vi "Configure Offset.vi"(8 "error in (no error)":errorcluster, 10 "offset":u16, 11 "TroSpec in":refnum<class "PL ISTEQ TroSpec.lvclass">) -> (0 "error out":errorcluster, 3 "TroSpec out":refnum<class "PL ISTEQ TroSpec.lvclass">)   [LabVIEW 2015, in "PL ISTEQ TroSpec.lvclass"]
doc: "Configures CCD offset."
uses:
  PL ISTEQ TroSpec.lvclass
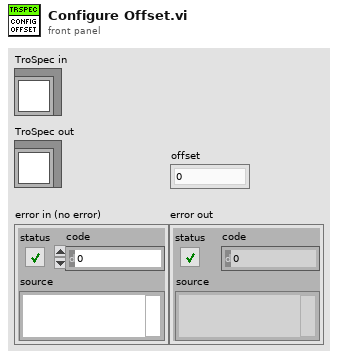
[diagram p1: front panel]
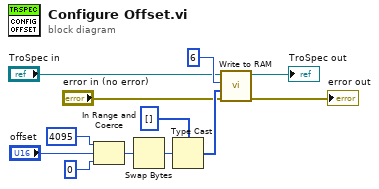
[diagram p0: block diagram]
diagram:
  n1 = In Range and Coerce(upper limit=u16 4095, x="offset", lower limit=u16 0) -> (coerced(x)=w3:u16)  [unwired: 1 out]
  n2 = Swap Bytes(anything=w3) -> (byte swapped=w5:u16)
  n3 = Type Cast(type=u8[] [] ("data"), x=w5) -> (*(type *) &x=w12:u8[])
  n4 = call "Write to RAM.vi"("error in (no error)"="error in (no error)", "data"=w12, "address"=u16 6, "TroSpec in"="TroSpec in") -> ("error out"=→"error out":errorcluster, "TroSpec out"=→"TroSpec out":refnum<class "PL ISTEQ TroSpec.lvclass">)  [unwired: 6 in]
